vi "Is Null Part.vi"(1 "Pattern Part":T1) -> (0 "Null Part":bool)   [LabVIEW 2020, in "Stream.lvlib" / "URLPattern.lvclass"]
uses:
  URLPattern.lvclass
  Pattern Part.ctl
  Pattern Part Type.ctl
  Pattern Part Modifier.ctl
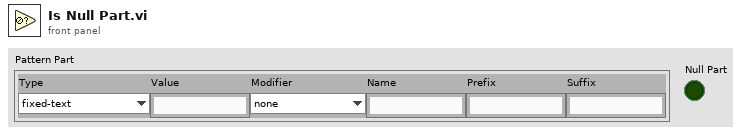
[diagram p1: front panel]
types:
  T1 = typedef "Stream.lvlib/URLPattern.lvclass/Pattern Part.ctl" = cluster{"Type":T2, "Value":string, "Modifier":T3, "Name":string, "Prefix":string, "Suffix":string}
  T2 = typedef "Stream.lvlib/URLPattern.lvclass/Pattern Part Type.ctl" = enum16{"fixed-text", "regexp", "segment-wildcard", "full-wildcard"}
  T3 = typedef "Stream.lvlib/URLPattern.lvclass/Pattern Part Modifier.ctl" = enum16{"none", "optional", "zero-or-more", "one-or-more"}
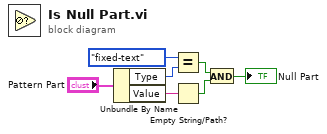
[diagram p0: block diagram]
diagram:
  n1 = Unbundle By Name("Pattern Part") -> ("Type"=w5:T2, "Value"=w7:string)
  n2 = Equal?(x=Pattern_Part_Type."fixed-text", y=w5) -> (x = y?=w3:bool)
  n3 = Empty String/Path?(string/path=w7) -> (empty?=w2:bool)
  n4 = And(x=w3, y=w2) -> (x .and. y?=→"Null Part":bool)
